vi "Stop Core.vi"(10 "final error code":i32, 11 "GarphView in":refnum<class "GarphView.lvclass">) -> (3 "GarphView out":refnum<class "GarphView.lvclass">)   [LabVIEW 2020, in "GarphView.lvlib" / "GarphView.lvclass"]
uses:
  GarphView.lvclass
  GarphView.lvclass/GarphView.ctl
  D:/Git/FATE-Platform/Executive/Interface/IExecutiveViews/IExecutiveViews/IExecutiveViews.lvclass
  <vilib>/gpm_packages/@cs/lookup-table/Source/LookupTable/LookupTable.lvclass
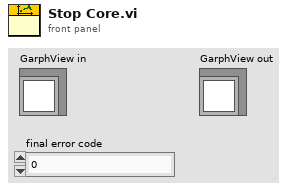
[diagram p1: front panel]
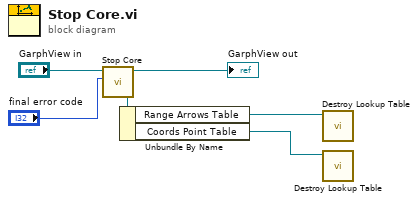
[diagram p0: block diagram]
diagram:
  n1 = call-parent "Stop Core.vi"("final error code"="final error code", "IViewable in"="GarphView in") -> ("IViewable out"=w3:refnum<class "GarphView.lvclass">)  [unwired: 9 in]
  "GarphView out" <- w3
  n2 = Unbundle By Name(w3) -> ("Range Arrows Table"=w2:refnum<data-value>, "Coords Point Table"=w1:refnum<data-value>)
  n3 = call <vilib>:"Destroy Lookup Table.vi"("LookupTable Reference"=w2) -> ()  [unwired: 10 in, 1 out]
  n4 = call <vilib>:"Destroy Lookup Table.vi"("LookupTable Reference"=w1) -> ()  [unwired: 10 in, 1 out]
